vi "Percent Error.vi"(1 "Measured Values":dbl, 2 "Accepted Value":dbl) -> (0 "Percent Error":dbl)   [LabVIEW 2016]
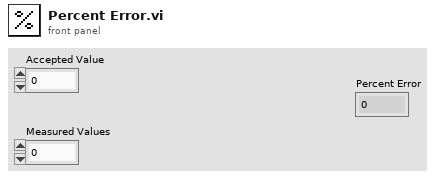
[diagram p1: front panel]
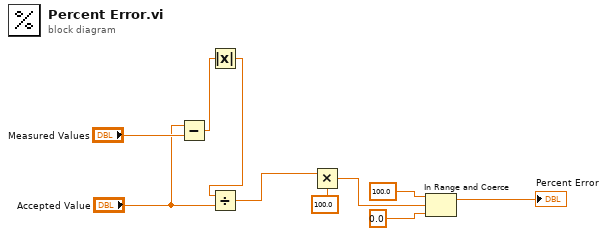
[diagram p0: block diagram]
diagram:
  n1 = Subtract(x="Accepted Value", y="Measured Values") -> (x-y=w2:dbl)
  n2 = Absolute Value(x=w2) -> (abs(x)=w1:dbl)
  n3 = Divide(x=w1, y="Accepted Value") -> (x/y=w8:dbl)
  n4 = Multiply(x=w8, y=100.0) -> (x*y=w4:dbl)
  n5 = In Range and Coerce(upper limit=100.0, x=w4, lower limit=0.0) -> (coerced(x)=→"Percent Error":dbl)  [unwired: 1 out]
